vi "Get Linker Errors Key Name.vi"() -> (2 "invalid namespace errors key":string, 3 "broken vis errors key":string)   [LabVIEW 2020, in "AB_Build.lvclass"]
uses:
  <vilib>/AppBuilder/AB_Classes/Build/AB_Build.lvclass
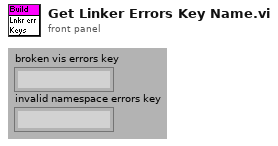
[diagram p1: front panel]
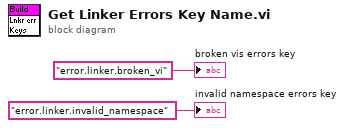
[diagram p0: block diagram]
diagram:
  "broken vis errors key" <- "error.linker.broken_vi" ("name")
  "invalid namespace errors key" <- "error.linker.invalid_namespace" ("name")
